vi "EventRegister.vi"(11 "SpectroscopyUI in":refnum<class "SpectroscopyUI.lvclass">) -> (3 "Event Registration Refnum":refnum<event-registration>)   [LabVIEW 2023, in "SpectroscopyUI.lvlib" / "SpectroscopyUI.lvclass"]
uses:
  SpectroscopyUI.lvclass
  SpectroscopyUI.lvclass/SpectroscopyUI.ctl
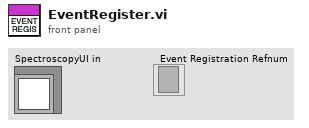
[diagram p1: front panel]
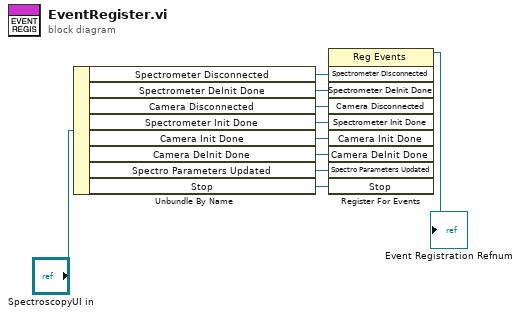
[diagram p0: block diagram]
diagram:
  n1 = Unbundle By Name("SpectroscopyUI in") -> ("Spectrometer Disconnected"=w3:refnum<user-event>, "Spectrometer DeInit Done"=w4:refnum<user-event>, "Camera Disconnected"=w5:refnum<user-event>, "Spectrometer Init Done"=w6:refnum<user-event>, "Camera Init Done"=w7:refnum<user-event>, "Camera DeInit Done"=w8:refnum<user-event>, "Spectro Parameters Updated"=w9:refnum<user-event>, "Stop"=w10:refnum<user-event>)
  n2 = register-events(w3, w4, w5, w6, w7, w8, w9, w10) -> (reference out=→"Event Registration Refnum":refnum<event-registration>)  [unwired: 2 in, 1 out]
